vi "MakeDataValuesOMFJSON.vi"(9 "Array of Values":string[](array[string]), 10 "OMF Dynamic Type Property Names and Formats":T1(array[cluster])=[{"Dynamic Property Name"="X acceleration", "Dynamic Property Format"=enum."string"}, {"Dynamic Property Name"="Y acceleration", "Dynamic Property Format"=enum."string"}, {"Dynamic Property Name"="Z acceleration", "Dynamic Property Format"=enum."string"}], 11 "OMF Container ID":string) -> (3 "OMF Data Values JSON":string)   [LabVIEW 2014]
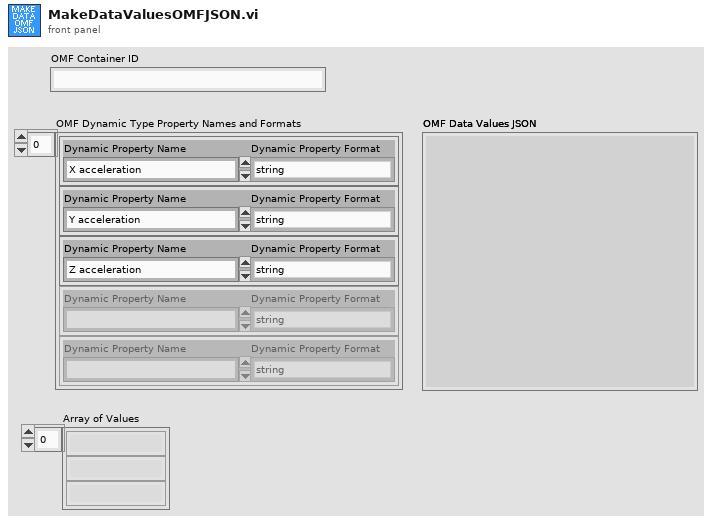
[diagram p1: front panel]
types:
  T1 = cluster{"Dynamic Property Name":string, "Dynamic Property Format":enum16{"string", "number"}}[]
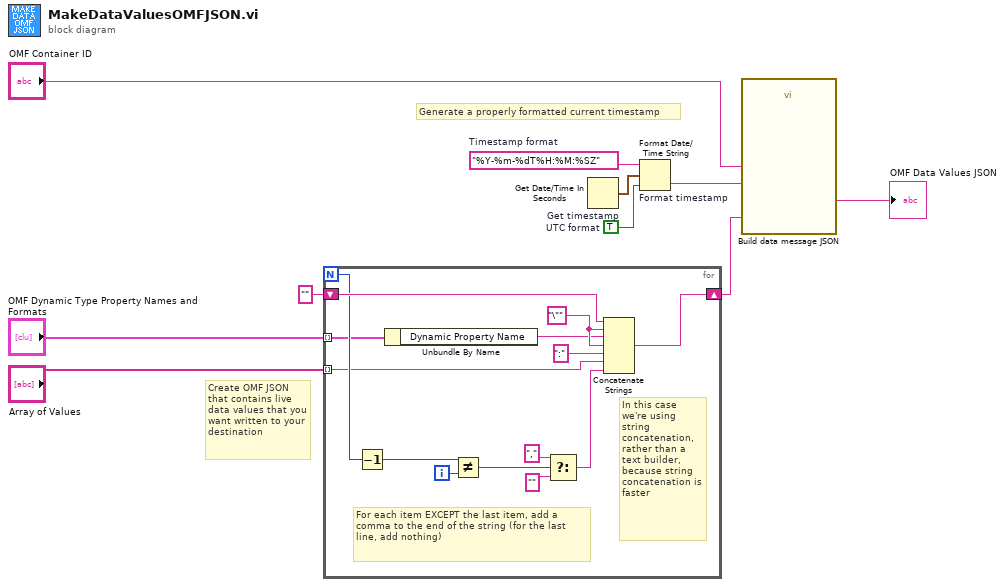
[diagram p0: block diagram]
diagram:
  w8 = TRUE  # UTC format
  w7 = "%Y-%m-%dT%H:%M:%SZ"  # Timestamp format
  # "Generate a properly formatted current timestamp"
  # "Create OMF JSON that contains live data values that you want written to your destination"
  n1 = for {
    N -> [w19]
    tunnel: "Array of Values" -> [w12] mode=indexing
    shift-right: [w24] -> w10
    shift-left: "" -> [w23]
    tunnel: "OMF Dynamic Type Property Names and Formats" -> [w14] mode=indexing
    i -> [w20]
    w21 = "\"" ("string")
    # "In this case we're using string concatenation, rather than a text builder, because string concatenation is faster"
    # "For each item EXCEPT the last item, add a comma to the end of the string (for the last line, add nothing)"
    n2 = Decrement(x=w19) -> (x-1=w18:i32)
    n3 = Unbundle By Name(w14) -> ("Dynamic Property Name"=w13:string)
    n4 = Not Equal?(x=w18, y=w20) -> (x != y?=w17:bool)
    n5 = Select(t="," ("string"), s=w17, f="") -> (s? t:f=w11:string)
    n6 = Concatenate Strings "Concatenate Strings"(w23, w21, w13, w21, ":" ("string"), w12, w11) -> (w24:string)
  }
  n7 = Get Date/Time In Seconds "Get timestamp"() -> (seconds since 1Jan1904=w9:timestamp)
  n8 = Format Date/Time String "Format timestamp"(time format string (%c)=w7, seconds (now)=w9, UTC format=w8) -> (date/time string=w6:string)
  n9 = call "Build data message JSON"("OMF Container ID"="OMF Container ID", "Timestamp"=w6, "Data Values Array"=w10) -> ("Result"=→"OMF Data Values JSON":string)  [unwired: 11 in, 1 out]
